vi "checkForceTriggerStiffnessTesting.vi"(8 "error in (no error)":errorcluster, 10 "Force Measured":dbl[unit]=1000000.0 min=1000000.0 max=300000000.0 format="%.1f", 11 "SystemController in":refnum<class "SystemController.lvclass">) -> (0 "error out":errorcluster, 2 "forceTriggerReached":bool, 3 "SystemController out":refnum<class "SystemController.lvclass">)   [LabVIEW 2015, in "SystemController.lvclass"]
uses:
  SystemController.lvclass
  SystemController.lvclass/SystemController.ctl
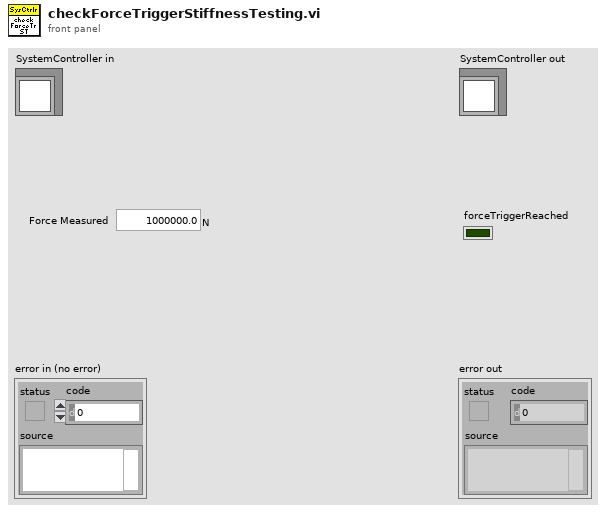
[diagram p1: front panel]
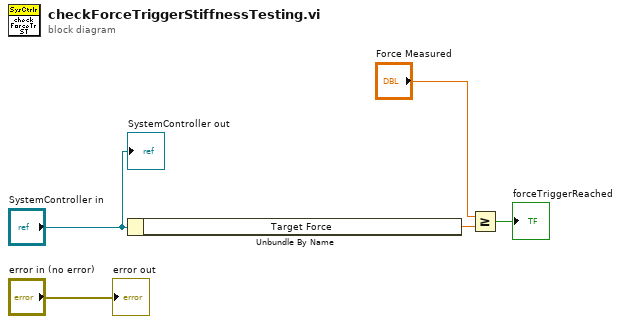
[diagram p0: block diagram]
diagram:
  n1 = Unbundle By Name("SystemController in") -> ("Target Force"=w2:dbl[unit])
  n2 = Greater Or Equal?(x="Force Measured", y=w2) -> (x >= y?=→"forceTriggerReached":bool)
  "error out" <- "error in (no error)"
  "SystemController out" <- "SystemController in"
